vi "Define Controls to Hide.vi"(6 "Troubleshooting Mode? (f)":bool, 8 "Show Calibration Values? (f)":bool, 9 "Other Controls to Hide":string[](array[string]), 10 "Measurement Information":T2={"Comments"="", "Directory Input"="", "Data file path"=path "C:/Data/EPR Data", "Scripting File"=path "C:/Data/Configuration Script.csv", "Save Data"=FALSE, "Tooth size (d11) [mm]"=0.0, "Tooth size (d12) [mm]"=0.0, "Tooth size (d21) [mm]"=0.0, "Tooth size (d22) [mm]"=0.0, "Dose of Tooth [Gy]"=0.0, "Safe Shutdown?"=FALSE, "Gases Available"=[], "Database Username"="", "Database Password"="", "Database Login URL"="", "Database Upload URL"="", "Database Success URL"="", "Database XML URL"="", "Database Resonator URL"="", "Session Number"=0, "Set #"=0, "Resonator Operator"="", "Session Type"="", "Tooth/Sample ID"="", "Volunteer ID"="", "Computer Operator"="", "Volunteer Type"="", "Site/Tooth Selection (T8,T9)"="", "Resonator"="", "Measurement Site"="", "Non-standard session?"=FALSE, "EPR DAQ Version"="", "Session Path"=path "C:/Data/EPR Data", "Chosen Applied State"="", "Chosen Initial State"="", "Time of Transition"="", "DAQ Mode"=enum."Engineering", "pO2/Scan [mmHg]"=[], "pO2/Set [mmHg]"=[], "Linewidth (HWHM)/Scan [Gauss]"=[], "Linewidth (HWHM)/Set [Gauss]"=[], "pO2 Conversion"="", "Dose Calibration Cluster"={"Dose Response"={"grand_mean"=0.0292016, "slope"=0.0188720543}, "Dose Correction"={"Sex"=1, "a0"=7.719669421, "a1"=-2.746550736, "a2"=-0.186490355, "a3"=0.041922063, "a4"=-0.849147359, "a5"=0.14330063, "a6"=0.019930219, "A_n"=40.0, "H_n"=10.12, "Dose Correction"=FALSE}, "Dose Reporting"={"Reporting is"=TRUE, "sd_threshold [AU]"=0.06, "sd_model [Gy]"=0.66, "dosimetric_threshold [Gy]"=2.0, "Add intrasession errors is"=FALSE, "Prior Radiation?"=FALSE}}, "OxyChip Slope"=0.0, "OxyChip Intercept"=0.0, "QA Mode"=enum."Select QA Mode", "QA Session?"=FALSE, "Sample Type"=enum."Empty Resonator", "Report pO2/Scan"=FALSE, "Skip End Session Save"=FALSE, "Number of sites"=enum."# Probes", "Recipient Name"="", "Sender Name"="", "Recipient Email"="", "Transition State History"=[], "pO2 Report Times"=[], "Temperature [C]"=0.0, "+Error pO2/Scan [mmHg]"=[], "-Error pO2/Scan [mmHg]"=[], "+Error pO2/Set [mmHg]"=[], "-Error pO2/Set [mmHg]"=[], "Oxy Phase Exclusion Tolerance [rad]"=0.0, "Oxy Center Exclusion Tolerance [%]"=0.0, "Oxy Exclude Unacceptable"=FALSE, "Oxy Unacceptable Estimate Flags"=[], "Save Session PPT"=FALSE, "Flagged Bad Sets"=[]} {"Oxy Center Exclusion Tolerance [%]" format="%#_9g"; "Oxy Phase Exclusion Tolerance [rad]" format="%#_9g"; "Temperature [C]" format="%#_9g"; "OxyChip Intercept" format="%#_9g"; "OxyChip Slope" format="%#_9g"; "Dose Calibration Cluster"."Dose Reporting"."dosimetric_threshold [Gy]" format="%#_9g"; "Dose Calibration Cluster"."Dose Reporting"."sd_model [Gy]" format="%#_9g"; "Dose Calibration Cluster"."Dose Reporting"."sd_threshold [AU]" format="%#_9g"; "Dose Calibration Cluster"."Dose Correction"."H_n" format="%#_9g"; "Dose Calibration Cluster"."Dose Correction"."A_n" format="%#_9g"; "Dose Calibration Cluster"."Dose Correction"."a6" format="%#.9g"; "Dose Calibration Cluster"."Dose Correction"."a5" format="%#.9g"; "Dose Calibration Cluster"."Dose Correction"."a4" format="%#.9g"; "Dose Calibration Cluster"."Dose Correction"."a3" format="%#.9g"; "Dose Calibration Cluster"."Dose Correction"."a2" format="%#.9g"; "Dose Calibration Cluster"."Dose Correction"."a1" format="%#.9g"; "Dose Calibration Cluster"."Dose Correction"."a0" format="%#.9g"; "Dose Calibration Cluster"."Dose Correction"."Sex" items=["Male"=1, "Female"=0]; "Dose Calibration Cluster"."Dose Response"."slope" format="%#_9g"; "Dose Calibration Cluster"."Dose Response"."grand_mean" format="%#_9g"}, 11 "Hardware Parameters":T1={"Scan Calibration [G/V]"=0.0, "Modulation Calibration [G/V]"=0.0, "Modulation Phase [deg]"=0.0, "Modulation Frequency [Hz]"=0.0, "Attenuation [dB]"=0, "Input Channel Count"=0, "Time constant"=7, "Sensitivity"=17, "Frequency Output Voltage [V]"=0.0, "Phase Output Voltage [V]"=0.0, "Lock-in Offset Compensation"=FALSE, "RF [GHz]"=0.0, "Q Start"=0.0, "Q End"=0.0, "Balance"=0.0, "Phase Error"=0.0, "AFC Error"=0.0, "AFC"=FALSE, "Magnet Rotation"=FALSE, "Balance Scaling Factor"=1.0, "Phase Error Scaling Factor"=1.0, "AFC Error Scaling Factor"=1.0, "Frequency Counter ID"="", "Sweep Waveform"=enum."Sawtooth", "Q-Factor Scale"=0.0, " Q-Data Scale"=0.0, " Q-Data Offset"=0.0, "Magnet Rotation Slope"=0.0, "Magnet Rotation Offset"=0.0, "Phase Sweep Resolution"=0.0, "Hardware Version Number"="", "Spectrometer ID Number"=0, "Spectrometer Name"="", "Lock in Saturation"=0.0, "Balance Threshold"=0.0, "Phase Error Threshold"=0.0, "AFC Error Threshold"=0.0, "Linear Actuator Length"=0.0, "Lock-in OK?"=FALSE, "Ignore Lock-in Comm. Failure"=FALSE, "Gradient Addresses"=[], "Gradient Calibrations [G/A*mm]"=[], "Gradient Power Supplies"=[], "Lock-in Address"="", "Magnet Type"=enum."RRI", "Camera Names"=[], "Sweep Limit [Gauss]"=0.0, "Modulation Limit [Gauss]"=0.0, "Balance Threshold Exceeded?"=FALSE, "Phase Threshold Exceeded?"=FALSE, "AFC Threshold Exceeded?"=FALSE, "Consecutive Re-tune attempts"=0, "Reverse Sweep Slope [sec]"=0.0, "Reverse Sweep Offset [G]"=0.0, "AFC Field Correction [V/MHz]"=0.0, "Active Gradients (X Y Z)"=[], "SpO2 Calibration [SpO2/V]"=1.0, "Heart Rate Calibration [BPM/V]"=1.0, "Thermocouple Channel"=""} {"Sensitivity" items=["", "2 nV", "5 nV", "10 nV", "20 nV", "50 nV", "100 nV", "200 nV", "500 nV", "1 uV", "2 uV", "5 uV", "10 uV", "20 uV", "50 uV", "100 uV", "200 uV", "500 uV", "1 mV", "2 mV", "5 mV", "10 mV", "20 mV", "50 mV", "100 mV", "200 mV", "500 mV", "1 V"]; "Time constant" items=["10 us", "20 us", "40 us", "80 us", "160 us", "320 us", "640 us", "5 ms", "10 ms", "20 ms", "50 ms", "100 ms", "200 ms", "500 ms", "1 s", "2 s", "5 s", "10 s", "20 s", "50 s", "100 s", "200 s", "500 s", "1 ks", "2 ks", "5 ks", "10 ks", "20 ks", "50 ks", "100 ks"]}) -> (3 "Controls to Hide":string[](array[string]))   [LabVIEW 2016]
uses:
  Types/Measurement Information.ctl
  Analysis/Dose Calculation and Reporting/Dose Calculation Control.ctl
  Types/Sample Type.ctl
  Types/Hardware Parameters.ctl
panel:
  # "Bridge I/O"
  # "Magnet Rotation"
  # "Field Calibration"
  # "Lock In Amplifier"
  # "Spectrometer Information"
  # "DAQ Settings"
  # "Gradient Coils and Field"
  # "X"
  # "Y"
  # "Z"
  # "Q-Measurements"
  # "Session Information"
  # "Oximetric Data and Information"
  # "Email"
  # "Tooth Information"
  # "Database"
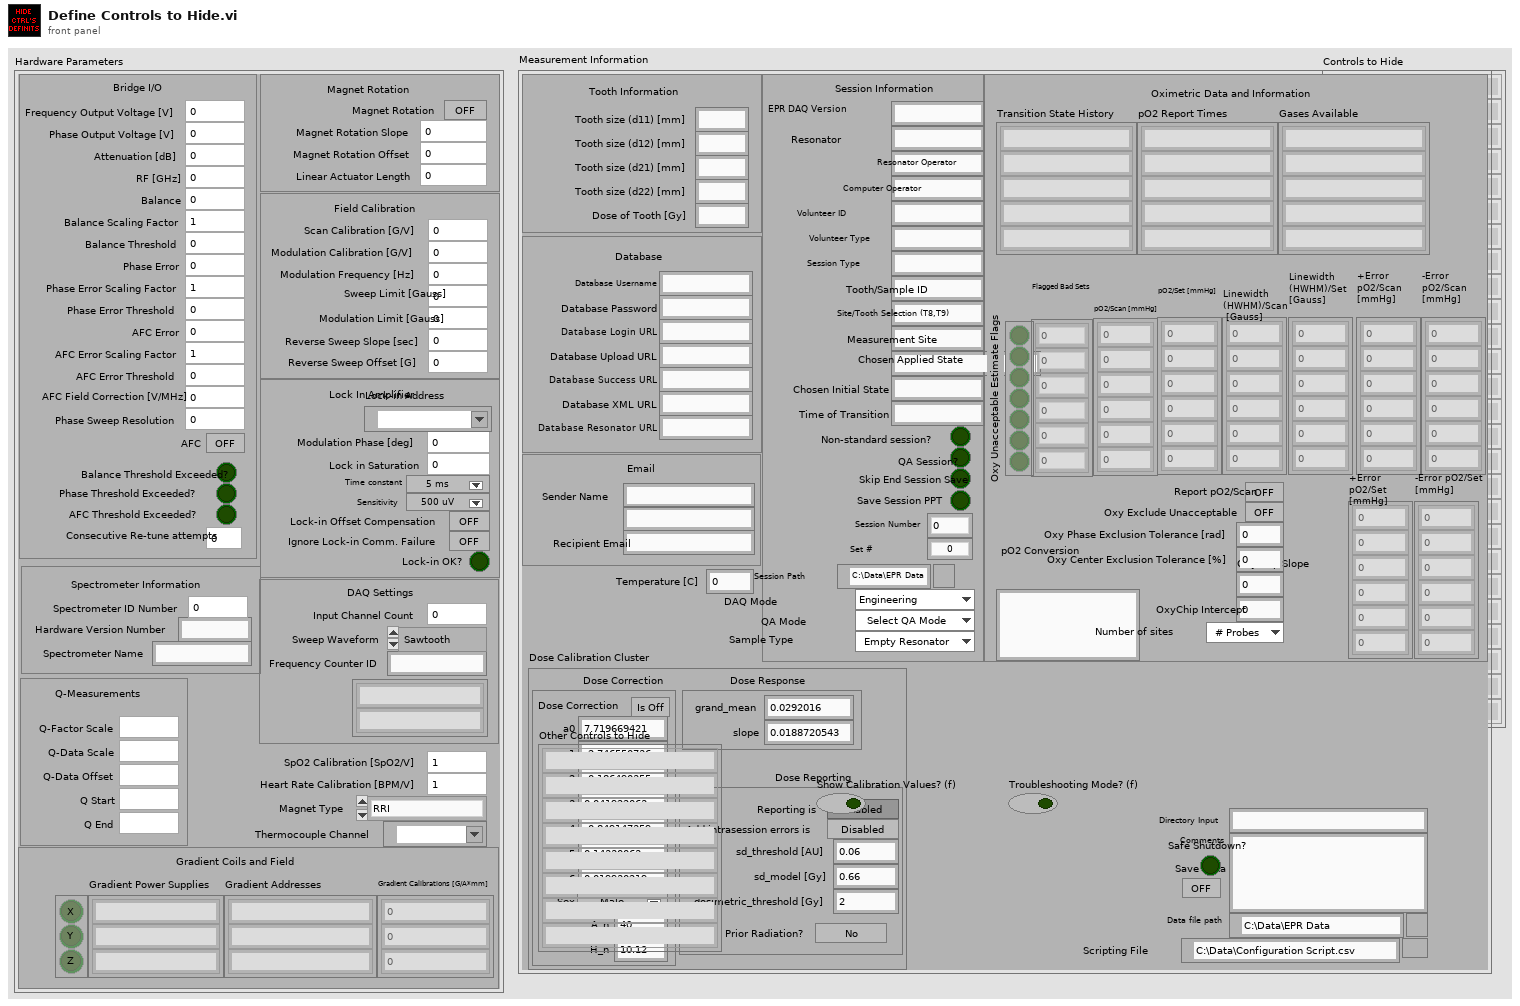
[diagram p1: front panel]
types:
  T1 = typedef "Hardware Parameters.ctl" = cluster{"Scan Calibration [G/V]":dbl, "Modulation Calibration [G/V]":dbl, "Modulation Phase [deg]":dbl, "Modulation Frequency [Hz]":dbl, "Attenuation [dB]":u16, "Input Channel Count":i32, "Time constant":u16, "Sensitivity":u16, "Frequency Output Voltage [V]":dbl, "Phase Output Voltage [V]":dbl, "Lock-in Offset Compensation":bool, "RF [GHz]":dbl, "Q Start":dbl, "Q End":dbl, "Balance":dbl, "Phase Error":dbl, "AFC Error":dbl, "AFC":bool, "Magnet Rotation":bool, "Balance Scaling Factor":dbl, "Phase Error Scaling Factor":dbl, "AFC Error Scaling Factor":dbl, "Frequency Counter ID":string, "Sweep Waveform":enum16{"Sine Wave", "Square Wave", "Sawtooth", "Triangle Wave"}, "Q-Factor Scale":dbl, " Q-Data Scale":dbl, " Q-Data Offset":dbl, "Magnet Rotation Slope":dbl, "Magnet Rotation Offset":dbl, "Phase Sweep Resolution":dbl, "Hardware Version Number":string, "Spectrometer ID Number":i32, "Spectrometer Name":string, "Lock in Saturation":dbl, "Balance Threshold":dbl, "Phase Error Threshold":dbl, "AFC Error Threshold":dbl, "Linear Actuator Length":dbl, "Lock-in OK?":bool, "Ignore Lock-in Comm. Failure":bool, "Gradient Addresses":string[], "Gradient Calibrations [G/A*mm]":dbl[], "Gradient Power Supplies":string[], "Lock-in Address":refnum<visa-resource-name>, "Magnet Type":enum16{"RRI", "BARDA", "Whole Body Permanent", "RRI Electromagnet"}, "Camera Names":string[], "Sweep Limit [Gauss]":dbl, "Modulation Limit [Gauss]":dbl, "Balance Threshold Exceeded?":bool, "Phase Threshold Exceeded?":bool, "AFC Threshold Exceeded?":bool, "Consecutive Re-tune attempts":i32, "Reverse Sweep Slope [sec]":dbl, "Reverse Sweep Offset [G]":dbl, "AFC Field Correction [V/MHz]":dbl, "Active Gradients (X Y Z)":bool[], "SpO2 Calibration [SpO2/V]":dbl, "Heart Rate Calibration [BPM/V]":dbl, "Thermocouple Channel":tag}
  T2 = typedef "Measurement Information.ctl" = cluster{"Comments":string, "Directory Input":string, "Data file path":path, "Scripting File":path, "Save Data":bool, "Tooth size (d11) [mm]":dbl, "Tooth size (d12) [mm]":dbl, "Tooth size (d21) [mm]":dbl, "Tooth size (d22) [mm]":dbl, "Dose of Tooth [Gy]":dbl, "Safe Shutdown?":bool, "Gases Available":string[], "Database Username":string, "Database Password":string, "Database Login URL":string, "Database Upload URL":string, "Database Success URL":string, "Database XML URL":string, "Database Resonator URL":string, "Session Number":i32, "Set #":u32, "Resonator Operator":string, "Session Type":string, "Tooth/Sample ID":string, "Volunteer ID":string, "Computer Operator":string, "Volunteer Type":string, "Site/Tooth Selection (T8,T9)":string, "Resonator":string, "Measurement Site":string, "Non-standard session?":bool, "EPR DAQ Version":string, "Session Path":path, "Chosen Applied State":string, "Chosen Initial State":string, "Time of Transition":string, "DAQ Mode":enum16{"Engineering", "Dosimetry", "Oximetry"}, "pO2/Scan [mmHg]":dbl[][], "pO2/Set [mmHg]":dbl[][], "Linewidth (HWHM)/Scan [Gauss]":dbl[][], "Linewidth (HWHM)/Set [Gauss]":dbl[][], "pO2 Conversion":string, "Dose Calibration Cluster":T3, "OxyChip Slope":dbl, "OxyChip Intercept":dbl, "QA Mode":enum16{"Select QA Mode", "QA-Start/End", "QA-Mid", "QA-Weekly", "QA-Eng", "Check Calibration"}, "QA Session?":bool, "Sample Type":T4, "Report pO2/Scan":bool, "Skip End Session Save":bool, "Number of sites":enum16{"# Probes", "1", "2", "3", "4"}, "Recipient Name":string, "Sender Name":string, "Recipient Email":string, "Transition State History":string[], "pO2 Report Times":string[], "Temperature [C]":dbl, "+Error pO2/Scan [mmHg]":dbl[][], "-Error pO2/Scan [mmHg]":dbl[][], "+Error pO2/Set [mmHg]":dbl[][], "-Error pO2/Set [mmHg]":dbl[][], "Oxy Phase Exclusion Tolerance [rad]":dbl, "Oxy Center Exclusion Tolerance [%]":dbl, "Oxy Exclude Unacceptable":bool, "Oxy Unacceptable Estimate Flags":bool[], "Save Session PPT":bool, "Flagged Bad Sets":u32[]}
  T3 = typedef "Dose Calculation Control.ctl" = cluster{"Dose Response":cluster{"grand_mean":dbl, "slope":dbl}, "Dose Correction":cluster{"Sex":u16, "a0":dbl, "a1":dbl, "a2":dbl, "a3":dbl, "a4":dbl, "a5":dbl, "a6":dbl, "A_n":dbl, "H_n":dbl, "Dose Correction":bool}, "Dose Reporting":cluster{"Reporting is":bool, "sd_threshold [AU]":dbl, "sd_model [Gy]":dbl, "dosimetric_threshold [Gy]":dbl, "Add intrasession errors is":bool, "Prior Radiation?":bool}}
  T4 = typedef "Sample Type.ctl" = enum16{"Empty Resonator", "IRS", "BallZero", "Irradiated Tooth", "Non-irradiated Tooth", "OxyChip", "LiPc", "PDT", "India Ink"}
  T5 = enum16{"RRI", "BARDA", "Whole Body Permanent", "RRI Electromagnet"}
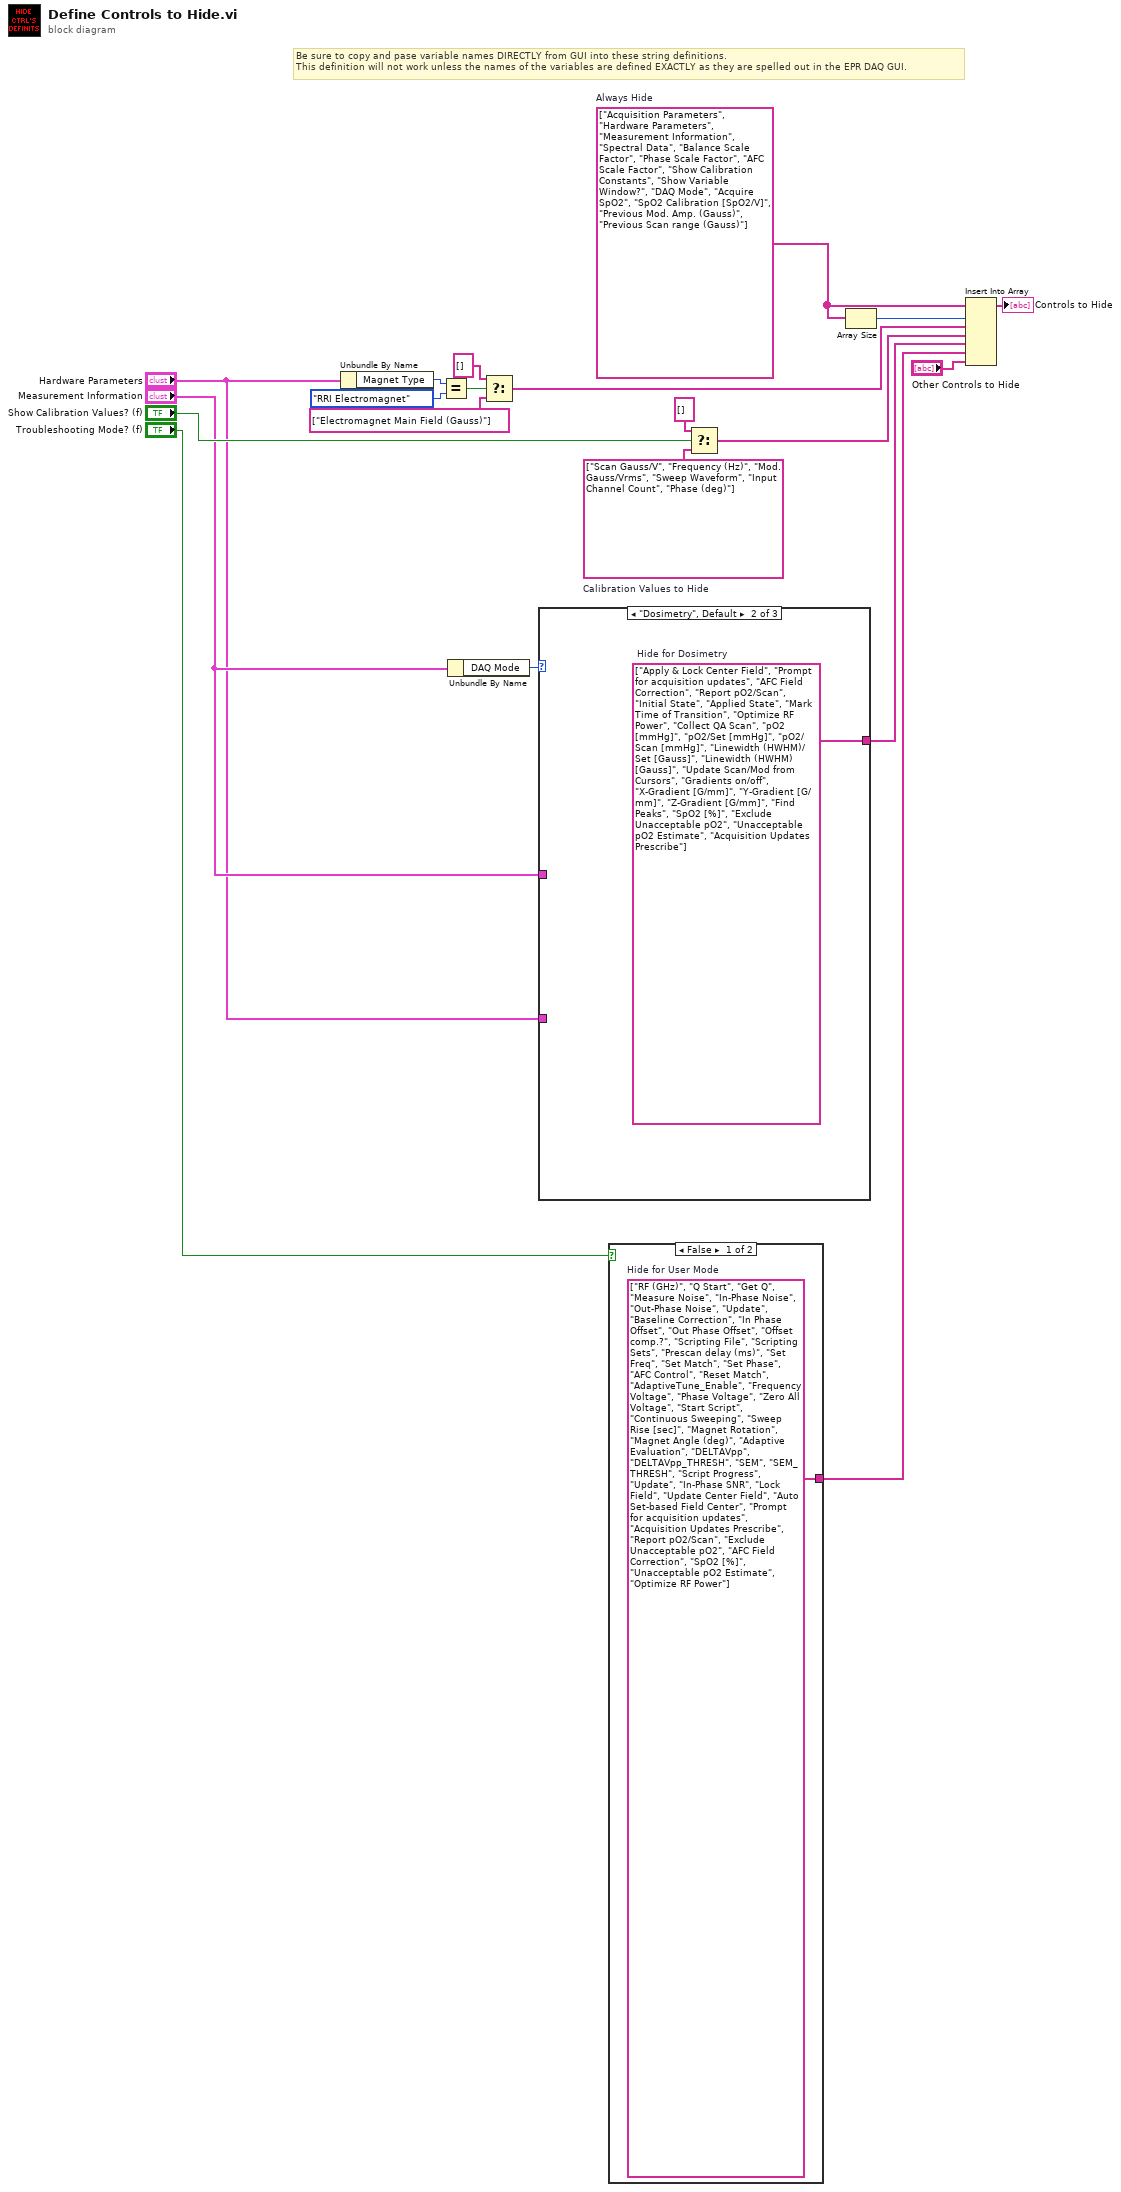
[diagram p0: block diagram]
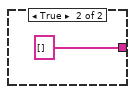
[diagram p2: hidden frame]
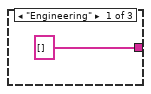
[diagram p3: hidden frame]
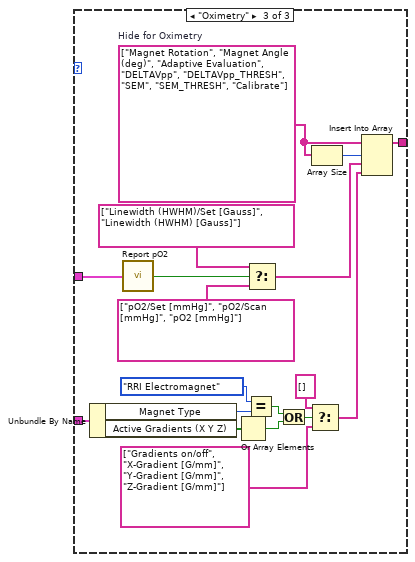
[diagram p4: hidden frame]
diagram:
  w13 = string[] ["Scan Gauss/V", "Frequency (Hz)", "Mod. Gauss/Vrms", "Sweep Waveform", "Input Channel Count", "Phase (deg)"]  # Calibration Values to Hide
  w19 = string[] ["Acquisition Parameters", "Hardware Parameters", "Measurement Information", "Spectral Data", "Balance Scale Factor", "Phase Scale Factor", "AFC Scale Factor", "Show Calibration Constants", "Show Variable Window?", "DAQ Mode", "Acquire SpO2", "SpO2 Calibration [SpO2/V]", "Previous Mod. Amp. (Gauss)", "Previous Scan range (Gauss)"]  # Always Hide
  # "Be sure to copy and pase variable names DIRECTLY from GUI into these string definitions.\nThis definition will not work unless the names of the variables are defined EXACTLY as they are spelled out in the EPR DAQ GUI."
  n1 = Unbundle By Name("Hardware Parameters") -> ("Magnet Type"=w16:T5)
  n2 = Equal?(x=w16, y=T5."RRI Electromagnet" ("Magnet Type")) -> (x = y?=w4:bool)
  n3 = Unbundle By Name("Measurement Information") -> ("DAQ Mode"=w17:enum16{"Engineering", "Dosimetry", "Oximetry"})
  n4 = Select(t=string[] [] ("Hide for Oximetry"), s=w4, f=string[] ["Electromagnet Main Field (Gauss)"] ("Hide for Oximetry")) -> (s? t:f=w14:string[])
  n5 = case shown="\"Dosimetry\", Default" w17 {
    tunnel: [string[] [] ("Hide for Oximetry") w22 w35] -> w1
    tunnel: "Measurement Information" -> [_ _ w40]
    tunnel: "Hardware Parameters" -> [_ _ w25]
    frame "Engineering" {
    }
    frame "Dosimetry", Default {
      w22 = string[] ["Apply & Lock Center Field", "Prompt for acquisition updates", "AFC Field Correction", "Report pO2/Scan", "Initial State", "Applied State", "Mark Time of Transition", "Optimize RF Power", "Collect QA Scan", "pO2 [mmHg]", "pO2/Set [mmHg]", "pO2/Scan [mmHg]", "Linewidth (HWHM)/Set [Gauss]", "Linewidth (HWHM) [Gauss]", "Update Scan/Mod from Cursors", "Gradients on/off", "X-Gradient [G/mm]", "Y-Gradient [G/mm]", "Z-Gradient [G/mm]", "Find Peaks", "SpO2 [%]", "Exclude Unacceptable pO2", "Unacceptable pO2 Estimate", "Acquisition Updates Prescribe"]  # Hide for Dosimetry
    }
    frame "Oximetry" {
      w34 = string[] ["Magnet Rotation", "Magnet Angle (deg)", "Adaptive Evaluation", "DELTAVpp", "DELTAVpp_THRESH", "SEM", "SEM_THRESH", "Calibrate"]  # Hide for Oximetry
      n6 = Unbundle By Name(w25) -> ("Magnet Type"=w30:T5, "Active Gradients (X Y Z)"=w24:bool[])
      n7 = call "Report pO2.vi"("Measurement Information"=w40) -> ("Report pO2"=w39:bool)
      n8 = Or Array Elements(Boolean array=w24) -> (logical OR=w23:bool)
      n9 = Equal?(x=T5."RRI Electromagnet" ("Magnet Type"), y=w30) -> (x = y?=w31:bool)
      n10 = Select(t=string[] ["Linewidth (HWHM)/Set [Gauss]", "Linewidth (HWHM) [Gauss]"] ("Hide for Oximetry"), s=w39, f=string[] ["pO2/Set [mmHg]", "pO2/Scan [mmHg]", "pO2 [mmHg]"] ("Hide for Oximetry")) -> (s? t:f=w36:string[])
      n11 = Or(x=w31, y=w23) -> (x .or. y?=w28:bool)
      n12 = Select(t=string[] [] ("Hide for Oximetry"), s=w28, f=string[] ["Gradients on/off", "X-Gradient [G/mm]", "Y-Gradient [G/mm]", "Z-Gradient [G/mm]"]) -> (s? t:f=w26:string[])
      n13 = Array Size(array=w34) -> (size(s)=w33:i32)
      n14 = Insert Into Array(array=w34, index=w33, new element #1=w36, new element #2=w26) -> (w35:string[])
    }
  }
  n15 = case shown="False" "Troubleshooting Mode? (f)" {
    tunnel: [w41 string[] [] ("Hide for Oximetry")] -> w5
    frame False {
      w41 = string[] ["RF (GHz)", "Q Start", "Get Q", "Measure Noise", "In-Phase Noise", "Out-Phase Noise", "Update", "Baseline Correction", "In Phase Offset", "Out Phase Offset", "Offset comp.?", "Scripting File", "Scripting Sets", "Prescan delay (ms)", "Set Freq", "Set Match", "Set Phase", "AFC Control", "Reset Match", "AdaptiveTune_Enable", "Frequency Voltage", "Phase Voltage", "Zero All Voltage", "Start Script", "Continuous Sweeping", "Sweep Rise [sec]", "Magnet Rotation", "Magnet Angle (deg)", "Adaptive Evaluation", "DELTAVpp", "DELTAVpp_THRESH", "SEM", "SEM_THRESH", "Script Progress", "Update", "In-Phase SNR", "Lock Field", "Update Center Field", "Auto Set-based Field Center", "Prompt for acquisition updates", "Acquisition Updates Prescribe", "Report pO2/Scan", "Exclude Unacceptable pO2", "AFC Field Correction", "SpO2 [%]", "Unacceptable pO2 Estimate", "Optimize RF Power"]  # Hide for User Mode
    }
    frame True {
    }
  }
  n16 = Select(t=string[] [] ("Hide for Oximetry"), s="Show Calibration Values? (f)", f=w13) -> (s? t:f=w2:string[])
  n17 = Array Size(array=w19) -> (size(s)=w20:i32)
  n18 = Insert Into Array(array=w19, index=w20, new element #1=w14, new element #2=w2, new element #3=w1, new element #4=w5, new element #5="Other Controls to Hide") -> (→"Controls to Hide":string[])
